vi "Remove Duplicates In Ftiness Values.vi"(11 "Random Numbers Array":u16[](array[numeric])=[762, 762, 762, 762, 760, 760, 765]) -> (3 "Random Numbers Array without Duplicates":u16[](array[numeric]))   [LabVIEW 2013]
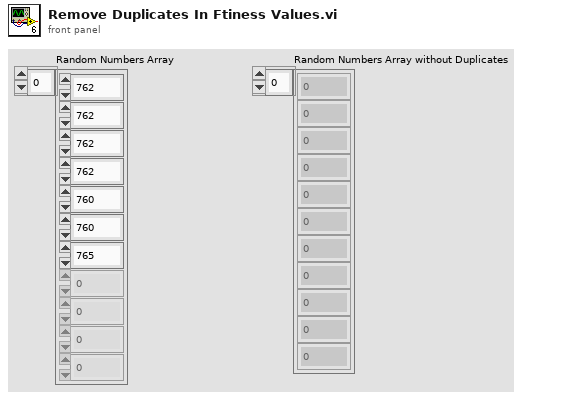
[diagram p1: front panel]
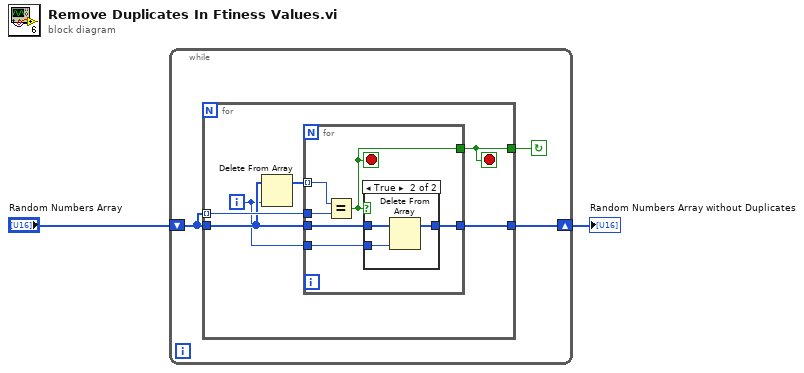
[diagram p0: block diagram]
diagram:
  n1 = while {
    shift-right: [w3] -> w1
    shift-left: "Random Numbers Array" -> [w5]
    stop <- w4 continue-if-true
    n2 = for {
      tunnel: w5 -> [w10] mode=indexing
      tunnel: w5 -> [w9]
      tunnel: [w7] -> w3
      tunnel: [w6] -> w4
      i -> [w8]
      stop <- w6 stop-if-true
      n3 = Delete From Array(array=w9, index=w8) -> (array with subset deleted=w11:u16[])  [unwired: 1 in, 1 out]
      n4 = for {
        tunnel: w11 -> [w17] mode=indexing
        tunnel: w10 -> [w16]
        tunnel: w9 -> [w15]
        tunnel: w8 -> [w14]
        tunnel: [w13] -> w7
        tunnel: [w12] -> w6
        stop <- w12 stop-if-true
        n5 = Equal?(x=w17, y=w16) -> (x = y?=w12:bool)
        n6 = case shown="True" w12 {
          tunnel: w15 -> [w18 w21]
          tunnel: w14 -> [_ w19]
          tunnel: [w18 w20] -> w13
          frame False {
          }
          frame True {
            n7 = Delete From Array(array=w21, index=w19) -> (array with subset deleted=w20:u16[])  [unwired: 1 in, 1 out]
          }
        }
      }
    }
  }
  "Random Numbers Array without Duplicates" <- w1
